vi "Array Gradient.vi"(7 "2D Array":dbl[][](array[numeric])) -> (4 "Gx (rows)":dbl[][](array[numeric]), 15 "Gy (col)":dbl[][](array[numeric]))   [LabVIEW 2020]
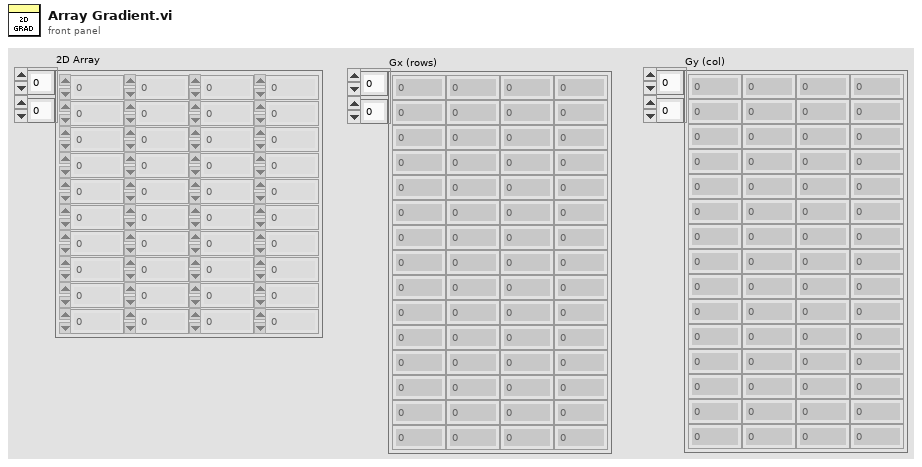
[diagram p1: front panel]
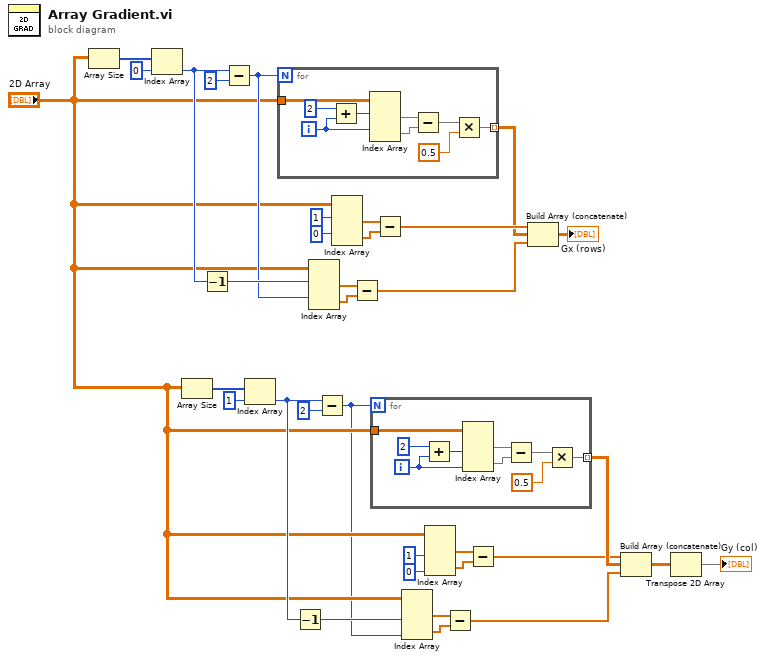
[diagram p0: block diagram]
diagram:
  n1 = Array Size(array="2D Array") -> (size(s)=w34:i32[])
  n2 = Index Array(array=w34, index=0) -> (element=w21:i32)
  n3 = Array Size(array="2D Array") -> (size(s)=w8:i32[])
  n4 = Decrement(x=w21) -> (x-1=w20:i32)
  n5 = Subtract(x=w21, y=2) -> (x-y=w19:i32)
  n6 = Index Array(array=w8, index=1) -> (element=w18:i32)
  n7 = for {
    N: w19 -> [_]
    tunnel: "2D Array" -> [w43]
    tunnel: [w36] -> w26 mode=indexing
    i -> [w42]
    n8 = Add(x=2, y=w42) -> (x+y=w35:i32)
    n9 = Index Array(array=w43, index (row) #1=w35, index (row) #2=w42) -> (element #1=w40:dbl[], element #2=w39:dbl[])  [unwired: 2 in]
    n10 = Subtract(x=w40, y=w39) -> (x-y=w38:dbl[])
    n11 = Multiply(x=w38, y=0.5) -> (x*y=w36:dbl[])
  }
  n12 = Decrement(x=w18) -> (x-1=w4:i32)
  n13 = Index Array(array="2D Array", index (row) #1=w20, index (row) #2=w19) -> (element #1=w23:dbl[], element #2=w24:dbl[])  [unwired: 2 in]
  n14 = Subtract(x=w18, y=2) -> (x-y=w3:i32)
  n15 = Index Array(array="2D Array", index (row) #1=1 ("index (row)"), index (row) #2=0 ("index (row)")) -> (element #1=w31:dbl[], element #2=w28:dbl[])  [unwired: 2 in]
  n16 = Subtract(x=w23, y=w24) -> (x-y=w22:dbl[])
  n17 = for {
    N: w3 -> [_]
    tunnel: "2D Array" -> [w52]
    tunnel: [w46] -> w14 mode=indexing
    i -> [w44]
    n18 = Add(x=2, y=w44) -> (x+y=w45:i32)
    n19 = Index Array(array=w52, index (col) #1=w45, index (col) #2=w44) -> (element #1=w50:dbl[], element #2=w49:dbl[])  [unwired: 2 in]
    n20 = Subtract(x=w50, y=w49) -> (x-y=w48:dbl[])
    n21 = Multiply(x=w48, y=0.5) -> (x*y=w46:dbl[])
  }
  n22 = Subtract(x=w31, y=w28) -> (x-y=w27:dbl[])
  n23 = Index Array(array="2D Array", index (col) #1=w4, index (col) #2=w3) -> (element #1=w16:dbl[], element #2=w15:dbl[])  [unwired: 2 in]
  n24 = Index Array(array="2D Array", index (col) #1=1 ("index (row)"), index (col) #2=0 ("index (row)")) -> (element #1=w11:dbl[], element #2=w12:dbl[])  [unwired: 2 in]
  n25 = Subtract(x=w16, y=w15) -> (x-y=w17:dbl[])
  n26 = Subtract(x=w11, y=w12) -> (x-y=w13:dbl[])
  n27 = Build Array (concatenate)(w27, w26, w22) -> (→"Gx (rows)":dbl[][])
  n28 = Build Array (concatenate)(w13, w14, w17) -> (w2:dbl[][])
  n29 = Transpose 2D Array(2D array=w2) -> (transposed array=→"Gy (col)":dbl[][])
